vi "Copy Set Default Value - Multiple Converter.vi"(11 "error in":errorcluster) -> (15 "error out":errorcluster)   [LabVIEW 2021, in "Converter.lvlib"]
uses:
  Converter.lvlib
  Path Functions/Path Functions.lvlib
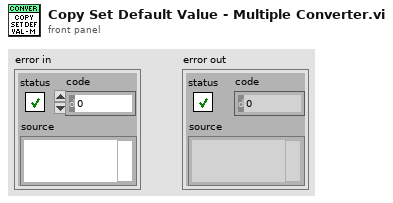
[diagram p1: front panel]
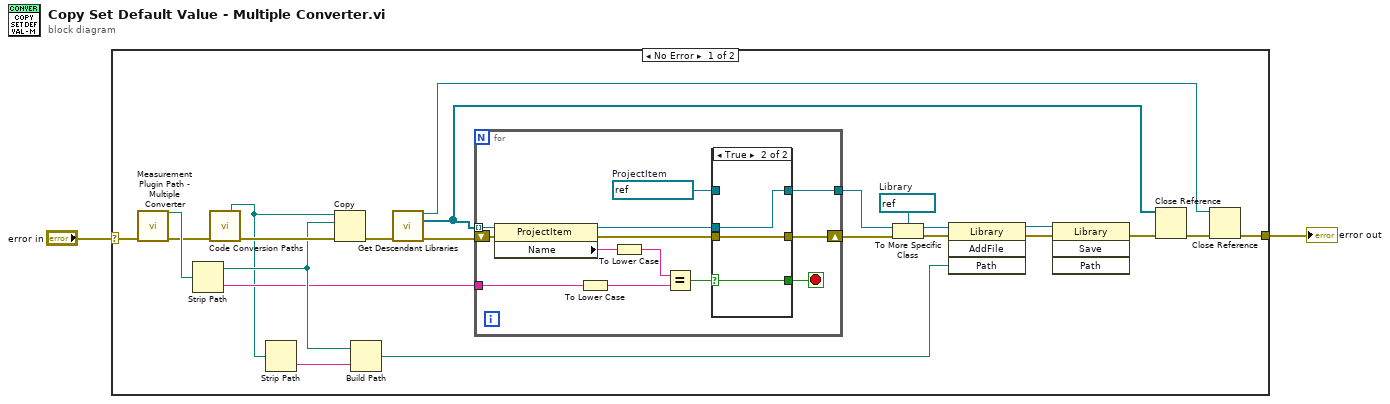
[diagram p0: block diagram]
diagram:
  n1 = case shown="No Error" "error in" {
    selector: "error in" -> [w12 w45]
    tunnel: [w16 w45] -> w2
    frame No Error {
      w5 = refnum<vi> refnum  # Library
      n2 = call "Measurement Plugin Path - Multiple Converter.vi"("error in"=w12) -> ("measurement ui lib"=w13:path, "error out"=w11:errorcluster)  [unwired: 2 in, 11 out]
      n3 = Strip Path(path=w13) -> (stripped path=w23:path, name=w22:string)
      n4 = call "Code Conversion Paths.vi"("error in"=w11) -> ("deafult value setter vi"=w15:path, "error out"=w25:errorcluster)  [unwired: 6 in, 7 out]
      n5 = Strip Path(path=w15) -> (name=w14:string)  [unwired: 1 out]
      n6 = Copy(8:w25, 10:w23, 11:w15) -> (0:w10:errorcluster)  [unwired: 2 in, 2 out]
      n7 = Build Path(base path=w23, name or relative path=w14) -> (appended path=w7:path)
      n8 = call "Get Descendant Libraries.vi"("error in"=w10) -> ("project out"=w17:refnum<vi>, "all descendents"=w21:refnum<vi>[], "error out"=w24:errorcluster)  [unwired: 12 in]
      n9 = for {
        tunnel: w21 -> [w38] mode=indexing
        tunnel: [w31] -> w19
        tunnel: w22 -> [w30]
        shift-right: [w26] -> w3
        shift-left: w24 -> [w29]
        stop <- w32 stop-if-true
        w35 = refnum<vi> refnum  # ProjectItem
        n10 = property class="ProjectItem"(reference=w38, error in=w29) -> (reference out=w34:refnum<vi>, error out=w33:errorcluster, "Name"=w37:string)
        n11 = To Lower Case(string=w30) -> (all lower case string=w27:string)
        n12 = To Lower Case(string=w37) -> (all lower case string=w28:string)
        n13 = Equal?(x=w28, y=w27) -> (x = y?=w36:bool)
        n14 = case shown="True" w36 {
          selector: w36 -> [w40 w43]
          tunnel: w34 -> [_ w44]
          tunnel: [w39 w42] -> w26
          tunnel: [w41 w44] -> w31
          tunnel: w35 -> [w41 _]
          tunnel: [w40 w43] -> w32
          tunnel: w33 -> [w39 w42]
          frame False {
          }
          frame True {
          }
        }
      }
      n15 = To More Specific Class(target class=w5, reference=w19, error in=w3) -> (specific class reference=w4:refnum<vi>, error out=w6:errorcluster)
      n16 = invoke class="Library" method="AddFile"(reference=w4, error in=w6, "Path"=w7) -> (reference out=w9:refnum<vi>, error out=w8:errorcluster)  [unwired: 1 in, 2 out]
      n17 = invoke class="Library" method="Save"(reference=w9, error in=w8) -> (error out=w18:errorcluster)  [unwired: 2 in, 3 out]
      n18 = Close Reference(reference=w21, error in (no error)=w18) -> (error out=w20:errorcluster)
      n19 = Close Reference(reference=w17, error in (no error)=w20) -> (error out=w16:errorcluster)
    }
    frame Error {
    }
  }
  "error out" <- w2
